vi "MetaListBoxToJson.vi"(8 "error in (no error)":errorcluster, 11 "ref in 2":refnum<vi>) -> (0 "error out":errorcluster, 3 "JSON queue ou":string)   [LabVIEW 2019]
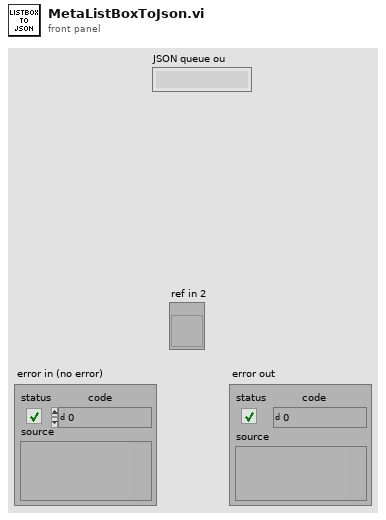
[diagram p1: front panel]
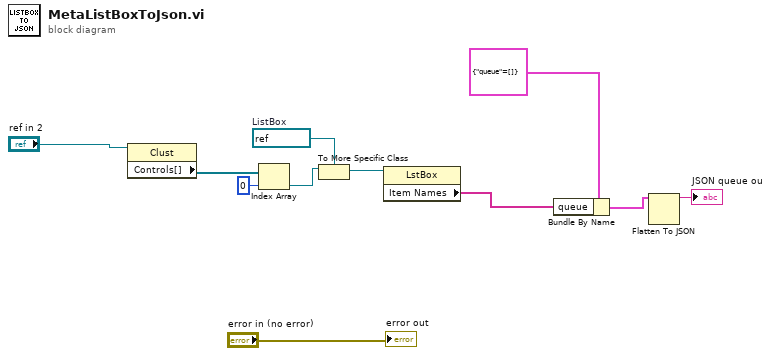
[diagram p0: block diagram]
diagram:
  w9 = refnum<vi> refnum  # ListBox
  n1 = property class="Clust"(reference="ref in 2") -> ("Controls[]"=w7:refnum<vi>[])  [unwired: 1 in, 2 out]
  n2 = Index Array(array=w7, index=0) -> (element=w10:refnum<vi>)
  n3 = To More Specific Class(target class=w9, reference=w10) -> (specific class reference=w8:refnum<vi>)  [unwired: 1 in, 1 out]
  n4 = property class="LstBox"(reference=w8) -> ("Item Names"=w1:string[])  [unwired: 1 in, 2 out]
  n5 = Bundle By Name(cluster=cluster{"queue":string[]} {"queue"=[]} ("input cluster"), "queue"=w1) -> (w3:cluster{"queue":string[]})
  n6 = Flatten To JSON(anything=w3) -> (JSON string=→"JSON queue ou":string)  [unwired: 2 in, 1 out]
  "error out" <- "error in (no error)"
